vi "From 1D Bool Tree Data.vi"(11 "Tree Data":refnum<class "Tree Data.lvclass">) -> (2 "1D Bool":bool[](array[boolean]))   [LabVIEW 2017, in "Tree API.lvlib" / "1D Bool.lvclass"]
doc: "Extract a 1D Bool value from Tree Data type."
uses:
  1D Bool.lvclass
  Tree Data/Tree Data.lvclass
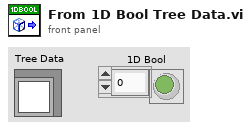
[diagram p1: front panel]
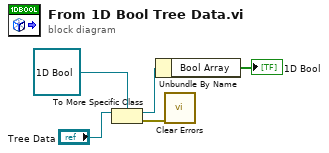
[diagram p0: block diagram]
diagram:
  n1 = To More Specific Class(target class=refnum<class "1D Bool.lvclass"> refnum ("Bool Array.lvclass"), reference="Tree Data") -> (specific class reference=w3:refnum<class "1D Bool.lvclass">, error out=w2:errorcluster)  [unwired: 1 in]
  n2 = Unbundle By Name(w3) -> ("Bool Array"=→"1D Bool":bool[])
  n3 = call <vilib>:"Clear Errors.vi"("error in (no error)"=w2) -> ()  [unwired: 5 in, 2 out]
